vi "PC 1.3 Bin 5 N.vi"(4 "State":i16=-1, 5 "Time":dbl format="%.2f", 6 "Sensor Values":dbl[](array[numeric]), 7 "Set Points":dbl[](array[numeric])=[0.0]) -> (0 "required data":T3={"Set Point names"=["Device ID"], "required number of setpoints"=1, "required number of sensors"=0, "Sensor names"=[]}, 3 "output value":dbl)   [LabVIEW 2019]
uses:
  modbusrtu/MB ID-Address.ctl
  modbusrtu/SerialParameters.ctl
  modbusrtu/MB cmd buffer.ctl
panel:
  in  "ChemTracChannels":string[](array[string])=["UV 1.1 UVA", "UV 1.1 UVT", "UV 1.1 Compensated UVA", "UV 1.1 COD", "UV 1.1 TOC", "PC 1.2 Cell ", "PC 1.2 Laser ", "PC 1.2 Total N", "PC 1.2 Bin 1 N", "PC 1.2 Bin 2 N", "PC 1.2 Bin 3 N", "PC 1.2 Bin 4 N", "PC 1.2 Bin 5 N", "PC 1.2 Bin 6 N", "PC 1.2 Total ppb", "PC 1.2 Bin 1 ppb", "PC 1.2 Bin 2 ppb", "PC 1.2 Bin 3 ppb", "PC 1.2 Bin 4 ppb", "PC 1.2 Bin 5 ppb", "PC 1.2 Bin 6 ppb", "PC 1.3 Cell ", "PC 1.3 Laser ", "PC 1.3 Total N", "PC 1.3 Bin 1 N", "PC 1.3 Bin 2 N", "PC 1.3 Bin 3 N", "PC 1.3 Bin 4 N", "PC 1.3 Bin 5 N", "PC 1.3 Bin 6 N", "PC 1.3 Total ppb", "PC 1.3 Bin 1 ppb", "PC 1.3 Bin 2 ppb", "PC 1.3 Bin 3 ppb", "PC 1.3 Bin 4 ppb", "PC 1.3 Bin 5 ppb", "PC 1.3 Bin 6 ppb"]
  in  "MB ID-Address in":T1
  # "Input Registers (Read Only)\nModbus Map: HydroAct 4 (75FC:4543:F24F:4856)\nAddress Size Type Device Description Ref.\n0 2 FLOAT UV-254 1.1 Official Value - UVA\n2 2 FLOAT UV-254 1.1 Official Value - UVT\n4 2 FLOAT UV-254 1.1 Official Value - Compensated UVA\n6 2 FLOAT UV-254 1.1 Official Value - COD\n8 2 FLOAT UV-254 1.1 Official Value - TOC\n10 2 FLOAT Particle Counter 1.2 Official Value - Cell\n12 2 FLOAT Particle Counter 1.2 Official Value - Laser\n14 2 FLOAT Particle Counter 1.2 Official Value - Total Counts\n16 2 FLOAT Particle Counter 1.2 Official Value - Counts Bin 1\n18 2 FLOAT Particle Counter 1.2 Official Value - Counts Bin 2\n20 2 FLOAT Particle Counter 1.2 Official Value - Counts Bin 3\n22 2 FLOAT Particle Counter 1.2 Official Value - Counts Bin 4\n24 2 FLOAT Particle Counter 1.2 Official Value - Counts Bin 5\n26 2 FLOAT Particle Counter 1.2 Official Value - Counts Bin 6\n28 2 FLOAT Particle Counter 1.2 Official Value - Total PPB\n30 2 FLOAT Particle Counter 1.2 Official Value - PPB Bin 1\n32 2 FLOAT Particle Counter 1.2 Official Value - PPB Bin 2\n34 2 FLOAT Particle Counter 1.2 Official Value - PPB Bin 3\n36 2 FLOAT Particle Counter 1.2 Official Value - PPB Bin 4\n38 2 FLOAT Particle Counter 1.2 Official Value - PPB Bin 5\n40 2 FLOAT Particle Counter 1.2 Official Value - PPB Bin 6\n42 2 FLOAT Particle Counter 1.3 Official Value - Cell\n44 2 FLOAT Particle Counter 1.3 Official Value - Laser\n46 2 FLOAT Particle Counter 1.3 Official Value - Total Counts\n48 2 FLOAT Particle Counter 1.3 Official Value - Counts Bin 1\n50 2 FLOAT Particle Counter 1.3 Official Value - Counts Bin 2\n52 2 FLOAT Particle Counter 1.3 Official Value - Counts Bin 3\n54 2 FLOAT Particle Counter 1.3 Official Value - Counts Bin 4\n56 2 FLOAT Particle Counter 1.3 Official Value - Counts Bin 5\n58 2 FLOAT Particle Counter 1.3 Official Value - Counts Bin 6\n60 2 FLOAT Particle Counter 1.3 Official Value - Total PPB\n62 2 FLOAT Particle Counter 1.3 Official Value - PPB Bin 1\n64 2 FLOAT Particle Counter 1.3 Official Value - PPB Bin 2\n66 2 FLOAT Particle Counter 1.3 Official Value - PPB Bin 3\n68 2 FLOAT Particle Counter 1.3 Official Value - PPB Bin 4\n70 2 FLOAT Particle Counter 1.3 Official Value - PPB Bin 5\n72 2 FLOAT Particle Counter 1.3 Official Value - PPB Bin 6"
  # "Enter the correct information for this control code in the required data structure below. Then make the current value default by right clicking on the border of the data structure. Select \"data operations\" and then select \"make current value default\". These values will be displayed by process controller."
  # "HydroACT has even parity by default."
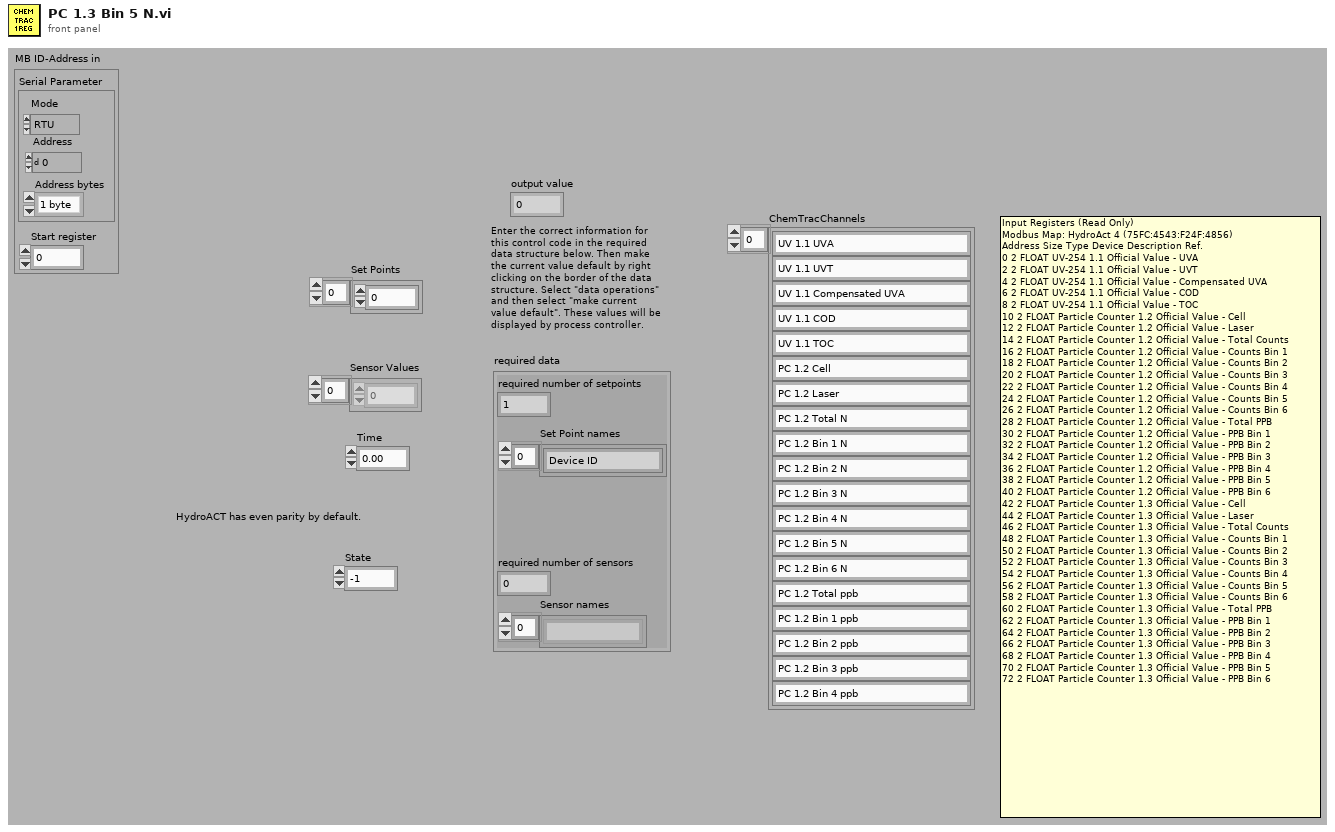
[diagram p1: front panel]
types:
  T1 = typedef "MB ID-Address.ctl" = cluster{"Serial Parameter":T2, "Start register":u16}
  T2 = typedef "SerialParameters.ctl" = cluster{"Mode":enum16{"RTU", "ASCII"}, "Address":u16, "Address bytes":enum16{"1 byte", "2 bytes"}}
  T3 = cluster{"Set Point names":string[], "required number of setpoints":u8, "required number of sensors":u8, "Sensor names":string[]}
  T4 = typedef "MB cmd buffer.ctl" = enum16{"ProCoDA", "MB succeed", "MB error", "MB Next Task", "ProCoDA read 1", "Commands pending"}
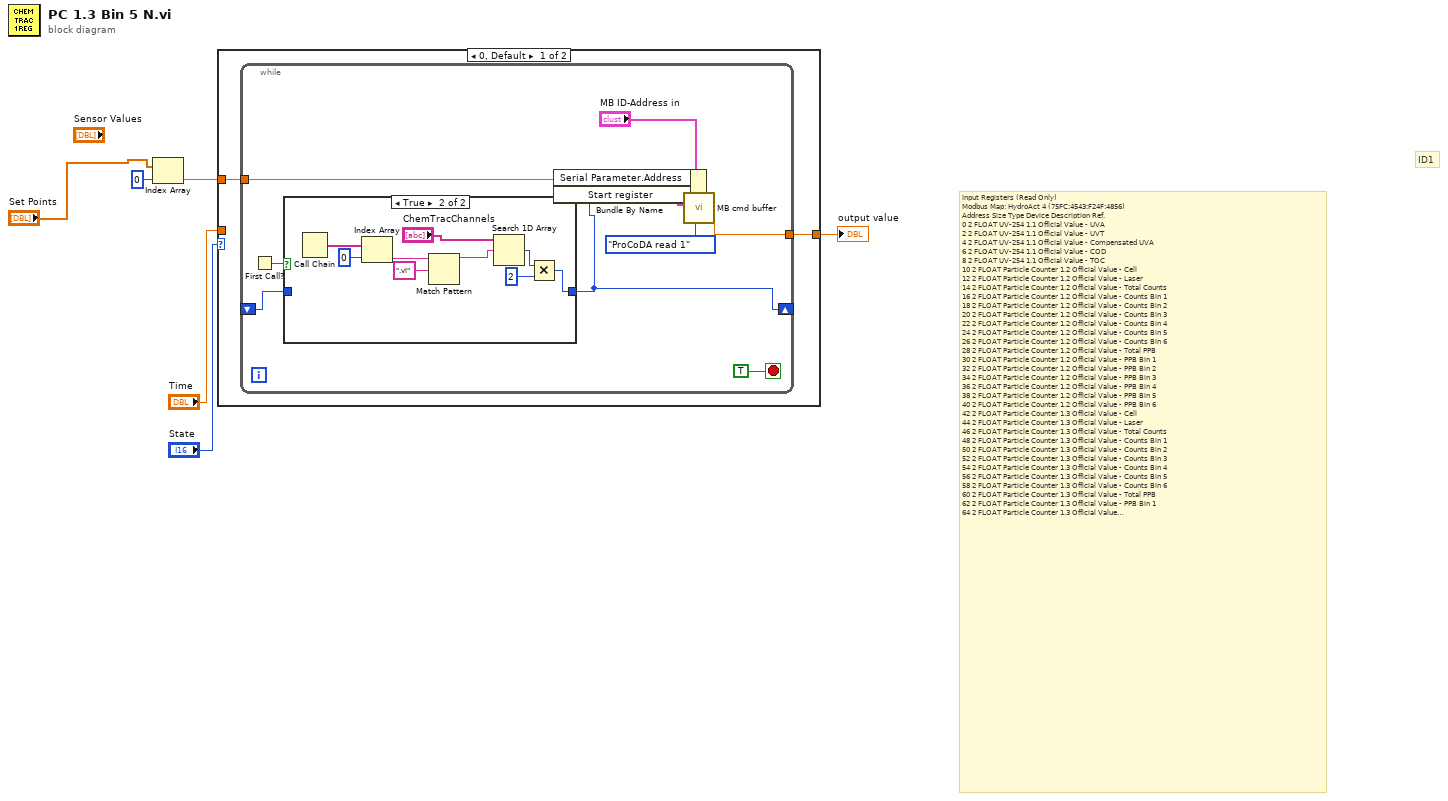
[diagram p0: block diagram]
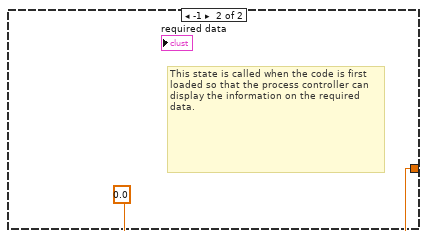
[diagram p3: hidden frame]
diagram:
  # "ID1"
  # "Input Registers (Read Only)\nModbus Map: HydroAct 4 (75FC:4543:F24F:4856)\nAddress Size Type Device Description Ref.\n0 2 FLOAT UV-254 1.1 Official Value - UVA\n2 2 FLOAT UV-254 1.1 Official Value - UVT\n4 2 FLOAT UV-254 1.1 Official Value - Compensated UVA\n6 2 FLOAT UV-254 1.1 Official Value - COD\n8 2 FLOAT UV-254 1.1 Official Value - TOC\n10 2 FLOAT Particle Counter 1.2 Official Value - Cell\n12 2 FLOAT Particle Counter 1.2 Official Value - Laser\n14 2 FLOAT Particle Counter 1.2 Official Value - Total Counts\n16 2 FLOAT Particle Counter 1.2 Official Value - Counts Bin 1\n18 2 FLOAT Particle Counter 1.2 Official Value - Counts Bin 2\n20 2 FLOAT Particle Counter 1.2 Official Value - Counts Bin 3\n22 2 FLOAT Particle Counter 1.2 Official Value - Counts Bin 4\n24 2 FLOAT Particle Counter 1.2 Official Value - Counts Bin 5\n26 2 FLOAT Particle Counter 1.2 Official Value - Counts Bin 6\n28 2 FLOAT Particle Counter 1.2 Official Value - Total PPB\n30 2 FLOAT Particle Counter 1.2 Official Value - PPB Bin 1\n32 2 FLOAT Particle Counter 1.2 Official Value - PPB Bin 2\n34 2 FLOAT Particle Counter 1.2 Official Value - PPB Bin 3\n36 2 FLOAT Particle Counter 1.2 Official Value - PPB Bin 4\n38 2 FLOAT Particle Counter 1.2 Official Value - PPB Bin 5\n40 2 FLOAT Particle Counter 1.2 Official Value - PPB Bin 6\n42 2 FLOAT Particle Counter 1.3 Official Value - Cell\n44 2 FLOAT Particle Counter 1.3 Official Value - Laser\n46 2 FLOAT Particle Counter 1.3 Official Value - Total Counts\n48 2 FLOAT Particle Counter 1.3 Official Value - Counts Bin 1\n50 2 FLOAT Particle Counter 1.3 Official Value - Counts Bin 2\n52 2 FLOAT Particle Counter 1.3 Official Value - Counts Bin 3\n54 2 FLOAT Particle Counter 1.3 Official Value - Counts Bin 4\n56 2 FLOAT Particle Counter 1.3 Official Value - Counts Bin 5\n58 2 FLOAT Particle Counter 1.3 Official Value - Counts Bin 6\n60 2 FLOAT Particle Counter 1.3 Official Value - Total PPB\n62 2 FLOAT Particle Counter 1.3 Official Value - PPB Bin 1\n64 2 FLOAT Particle Counter 1.3 Official Value - PPB Bin 2\n66 2 FLOAT Particle Counter 1.3 Official Value - PPB Bin 3\n68 2 FLOAT Particle Counter 1.3 Official Value - PPB Bin 4\n70 2 FLOAT Particle Counter 1.3 Official Value - PPB Bin 5\n72 2 FLOAT Particle Counter 1.3 Official Value - PPB Bin 6"
  n1 = Index Array(array="Set Points", index=0) -> (element=w2:dbl)
  n2 = case shown="0, Default" "State" {
    tunnel: [w8 0.0 ("fraction on")] -> w5
    tunnel: "Time" -> [_ _]
    tunnel: w2 -> [w7 _]
    frame 0, Default {
      n3 = while {
        tunnel: [w16] -> w8
        tunnel: w7 -> [w13]
        shift-right: [w11] -> _
        shift-left: _ -> [w10]
        stop <- TRUE stop-if-true
        n4 = First Call?() -> (First Call?: T/F=w12:bool)
        n5 = case shown="True" w12 {
          tunnel: [w18 w19] -> w11
          tunnel: w10 -> [w18 _]
          frame False {
          }
          frame True {
            n6 = Call Chain() -> (call chain=w26:string[])
            n7 = Index Array(array=w26, index=0) -> (element=w27:string)
            n8 = Match Pattern(string=w27, regular expression=".vi") -> (before substring=w22:string)  [unwired: 1 in, 3 out]
            n9 = Search 1D Array(1D array="ChemTracChannels", element=w22) -> (index of element=w21:i32)  [unwired: 1 in]
            n10 = Multiply(x=w21, y=2) -> (x*y=w19:i32)
          }
        }
        n11 = Bundle By Name(cluster="MB ID-Address in", "Serial Parameter.Address"=w13, "Start register"=w11) -> (w14:T1)
        n12 = call "MB cmd buffer.vi"("MB cmd buffer"=MB_cmd_buffer."ProCoDA read 1", "MB ID-Address in"=w14) -> ("output value"=w16:dbl)  [unwired: 3 in, 6 out]
      }
    }
    frame -1 {
      # "This state is called when the code is first loaded so that the process controller can display the information on the required data."
    }
  }
  "output value" <- w5
